vi "Frame Set Basic Data.vi"(8 "error in (no error)":errorcluster, 10 "Frame Basic Data":T1, 11 "IDE simple in":refnum<class "LF2R IDE.lvclass">) -> (0 "error out":errorcluster, 3 "IDE simple out":refnum<class "LF2R IDE.lvclass">)   [LabVIEW 2018, in "LF2R IDE.lvlib" / "LF2R IDE.lvclass"]
uses:
  LF2R IDE.lvclass
  Frame Analizer/frame basic data.ctl
  LF2R IDE.lvclass/LF2R IDE.ctl
  Frame Analizer/Data Parser.lvclass
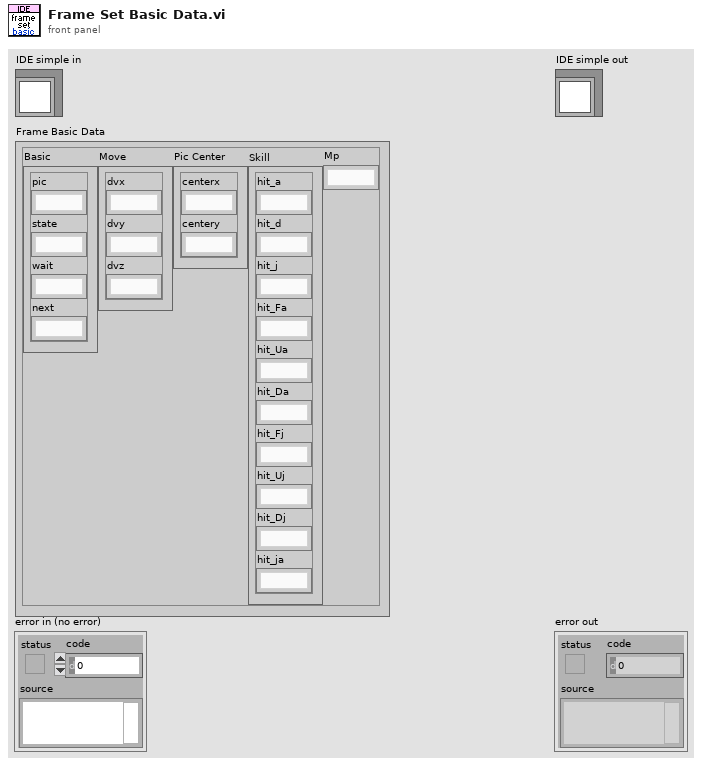
[diagram p1: front panel]
types:
  T1 = typedef "Data Parser.lvclass/frame basic data.ctl" = cluster{"Basic":cluster{"pic":string, "state":string, "wait":string, "next":string}, "Move":cluster{"dvx":string, "dvy":string, "dvz":string}, "Pic Center":cluster{"centerx":string, "centery":string}, "Skill":cluster{"hit_a":string, "hit_d":string, "hit_j":string, "hit_Fa":string, "hit_Ua":string, "hit_Da":string, "hit_Fj":string, "hit_Uj":string, "hit_Dj":string, "hit_ja":string}, "Mp":string}
  T2 = cluster{"pic":refnum<vi>, "state":refnum<vi>, "wait":refnum<vi>, "next":refnum<vi>}
  T3 = cluster{"centerx":refnum<vi>, "centery":refnum<vi>}
  T4 = cluster{"dvx":refnum<vi>, "dvy":refnum<vi>, "dvz":refnum<vi>}
  T5 = cluster{"hit_a":refnum<vi>, "hit_d":refnum<vi>, "hit_j":refnum<vi>, "hit_Fa":refnum<vi>, "hit_Ua":refnum<vi>, "hit_Da":refnum<vi>, "hit_Fj":refnum<vi>, "hit_Uj":refnum<vi>, "hit_Dj":refnum<vi>, "hit_ja":refnum<vi>}
  T6 = cluster{"pic":string, "state":string, "wait":string, "next":string}
  T7 = cluster{"dvx":string, "dvy":string, "dvz":string}
  T8 = cluster{"hit_a":string, "hit_d":string, "hit_j":string, "hit_Fa":string, "hit_Ua":string, "hit_Da":string, "hit_Fj":string, "hit_Uj":string, "hit_Dj":string, "hit_ja":string}
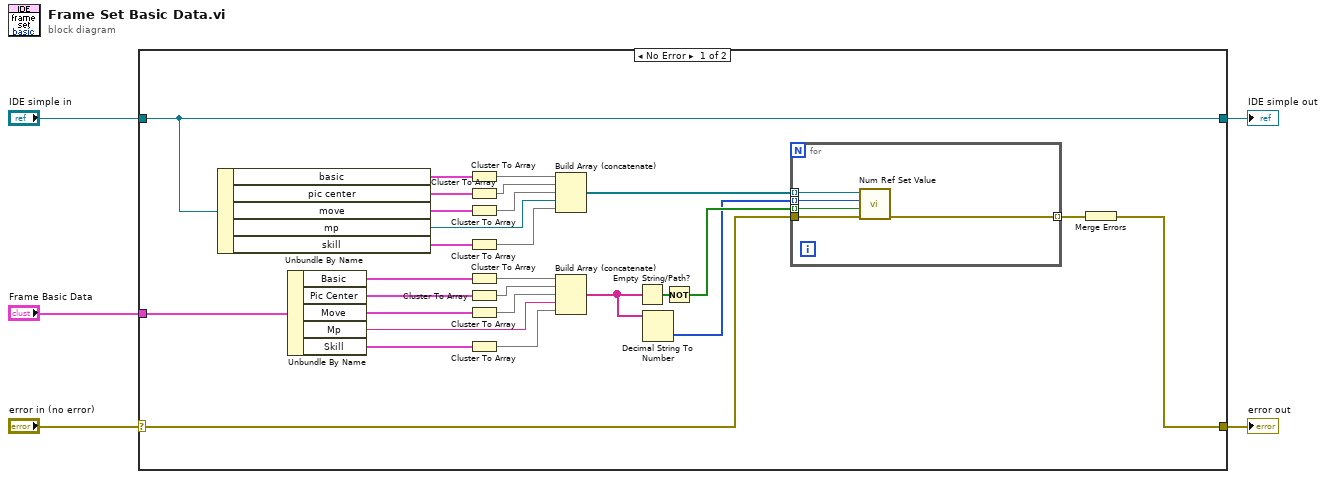
[diagram p0: block diagram]
diagram:
  n1 = case shown="No Error" "error in (no error)" {
    selector: "error in (no error)" -> [w30 w40]
    tunnel: [w6 w40] -> w4
    tunnel: [w8 w39] -> w2
    tunnel: "IDE simple in" -> [w8 w39]
    tunnel: "Frame Basic Data" -> [w31 _]
    frame No Error {
      n2 = Unbundle By Name(w8) -> ("basic"=w33:T2, "pic center"=w29:T3, "move"=w28:T4, "mp"=w23:refnum<vi>, "skill"=w27:T5)
      n3 = Unbundle By Name(w31) -> ("Basic"=w21:T6, "Pic Center"=w20:cluster{"centerx":string, "centery":string}, "Move"=w19:T7, "Mp"=w14:string, "Skill"=w18:T8)
      n4 = Cluster To Array(cluster=w33) -> (array=w26:refnum<vi>[])
      n5 = Cluster To Array(cluster=w29) -> (array=w25:refnum<vi>[])
      n6 = Cluster To Array(cluster=w28) -> (array=w24:refnum<vi>[])
      n7 = Cluster To Array(cluster=w27) -> (array=w22:refnum<vi>[])
      n8 = Cluster To Array(cluster=w21) -> (array=w17:string[])
      n9 = Cluster To Array(cluster=w20) -> (array=w16:string[])
      n10 = Cluster To Array(cluster=w19) -> (array=w15:string[])
      n11 = Cluster To Array(cluster=w18) -> (array=w13:string[])
      n12 = Build Array (concatenate)(w26, w25, w24, w23, w22) -> (w11:refnum<vi>[])
      n13 = Build Array (concatenate)(w17, w16, w15, w14, w13) -> (w12:string[])
      n14 = Empty String/Path?(string/path=w12) -> (empty?=w32:bool[])
      n15 = Decimal String To Number(string=w12) -> (number=w9:i32[])  [unwired: 2 in, 1 out]
      n16 = Not(x=w32) -> (.not. x?=w10:bool[])
      n17 = for {
        tunnel: w30 -> [w38]
        tunnel: w11 -> [w37] mode=indexing
        tunnel: w10 -> [w36] mode=indexing
        tunnel: w9 -> [w35] mode=indexing
        tunnel: [w34] -> w7 mode=indexing
        n18 = call "Num Ref Set Value.vi"("error in"=w38, "Valid"=w36, "Value"=w35, "Num Ref"=w37) -> ("error out"=w34:errorcluster)  [unwired: 7 in]
      }
      n19 = Merge Errors(w7) -> (w6:errorcluster)
    }
    frame Error {
    }
  }
  "error out" <- w4
  "IDE simple out" <- w2
